vi "Set Column Value.vi"(9 "Value":string, 10 "Column":i32, 11 "Empty Row":string[](array[string])) -> (3 "Array":string[](array[string]))   [LabVIEW 2020, in "Astemes_CSVReportPlugin.lvlib" / "TestStand Result Handler.lvclass"]
uses:
  TestStand Result Handler.lvclass
  TestStand Result Handler.lvclass/TestStand Result Handler.ctl
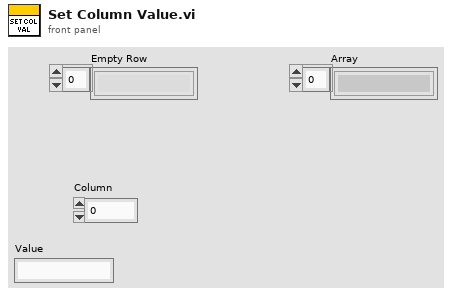
[diagram p1: front panel]
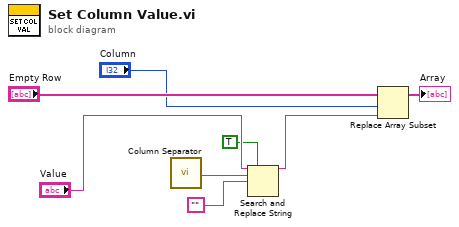
[diagram p0: block diagram]
diagram:
  n1 = call "Column Separator.vi"() -> ("delimiter"=w4:string)
  n2 = Search and Replace String(replace all?=TRUE ("replace all? (F)"), input string="Value", search string=w4, replace string="" ("replace string (\"\")")) -> (result string=w5:string)  [unwired: 4 in, 3 out]
  n3 = Replace Array Subset(array="Empty Row", new element=w5, index="Column") -> (→"Array":string[])
